vi "receiveTelemetry.vi"(8 "error in (no error)":errorcluster, 10 "Address":u32, 11 "FPGATelemetry in":refnum<class "FPGATelemetry.lvclass">) -> (0 "error out":errorcluster, 2 "Telemetry":u32, 3 "FPGATelemetry out":refnum<class "FPGATelemetry.lvclass">)   [LabVIEW 2015, in "FPGATelemetry.lvclass"]
uses:
  FPGATelemetry.lvclass
  FPGATelemetry.lvclass/FPGATelemetry.ctl
  <vilib>/Utility/error.llb/Error Cluster From Error Code.vi
  <vilib>/rvi/errors/niLvFpgaAdjustHostInterfaceError.vi
  <vilib>/rvi/interface/nirviMethod/nirviMethod.xnode
  <vilib>/FPGAPlugInAG/Dynamic/niLvFpga_WriteFifo_Dynamic.vi
  <vilib>/rvi/errors/niLvFpgaMergeErrorWithErrorCode.vi
  <vilib>/FPGAPlugInAG/Dynamic/niLvFpga_ReadFifo_Dynamic.vi
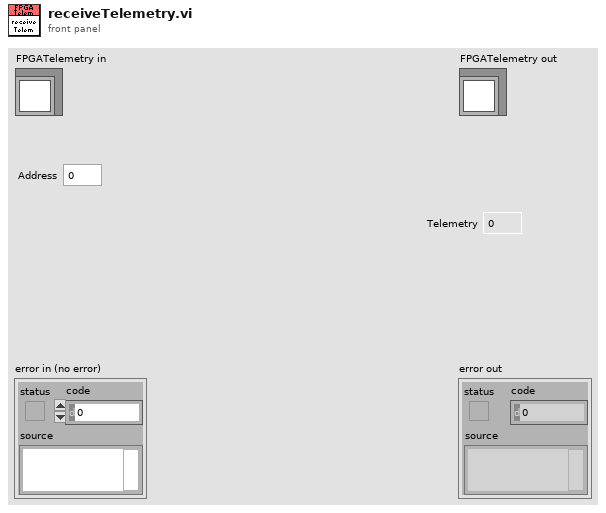
[diagram p1: front panel]
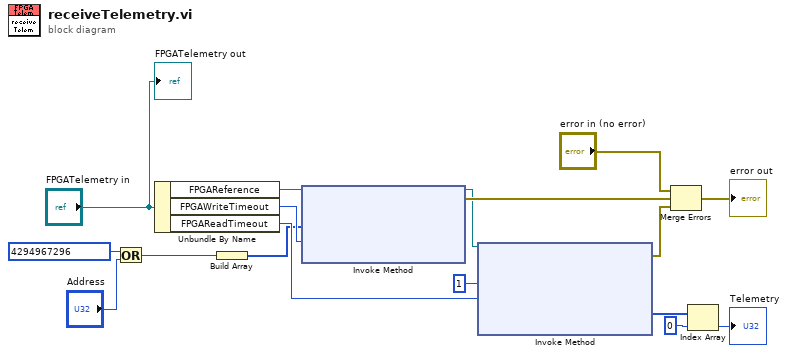
[diagram p0: block diagram]
diagram:
  n1 = Or(x=u64 4294967296, y="Address") -> (x .or. y?=w7:u64)
  n2 = Unbundle By Name("FPGATelemetry in") -> ("FPGAReference"=w17:refnum<k20>, "FPGAWriteTimeout"=w16:i32, "FPGAReadTimeout"=w15:i32)
  n3 = Build Array(w7) -> (w6:u64[])
  n4 = xnode "Invoke Method"("FPGA VI Reference In"=w17, "Data"=w6, "Timeout (ms)"=w16) -> ("FPGA VI Reference Out"=w4:refnum<k20>, "error out"=w13:errorcluster)  [unwired: 1 in, 1 out]
  n5 = xnode "Invoke Method"("FPGA VI Reference In"=w4, "Number of Elements"=u32 1, "Timeout (ms)"=w15) -> ("error out"=w12:errorcluster, "Data"=w3:u32[])  [unwired: 1 in, 2 out]
  n6 = Merge Errors("error in (no error)", w13, w12) -> (→"error out":errorcluster)
  n7 = Index Array(array=w3, index=0) -> (element=→"Telemetry":u32)
  "FPGATelemetry out" <- "FPGATelemetry in"
